vi "Register to IncomingMessages.vi"(8 "error in":errorcluster, 11 "Actor Class":T1) -> (0 "error out":errorcluster, 3 "Incoming Messages":refnum<event-registration>)   [LabVIEW 2013]
uses:
  Actor Private Data.ctl
  <vilib>/LabVIEW Open Source Project/MQTT Client/Client class/Client.lvclass
  Actor Private Events -- cluster.ctl
  Payload -- cluster.ctl
  <vilib>/LabVIEW Open Source Project/MQTT Client/Client class/Public Events -- cluster.ctl
  <vilib>/LabVIEW Open Source Project/MQTT Control Packets/Control Packets/CONNACK/Connect Return Code -- enum.ctl
  <vilib>/LabVIEW Open Source Project/MQTT Control Packets/Control Packets/PUBLISH/PUBLISH.lvclass
  <vilib>/LabVIEW Open Source Project/MQTT Client/Client class/Client.lvclass/Client.ctl
  <vilib>/LabVIEW Open Source Project/MQTT Control Packets/Control Packets/CONNACK/CONNACK.lvclass
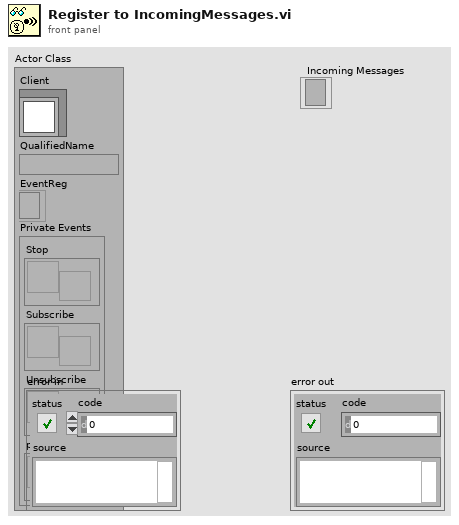
[diagram p1: front panel]
types:
  T1 = typedef "Actor Private Data.ctl" = cluster{"Client":refnum<class "Client.lvclass">, "QualifiedName":string, "EventReg":refnum<event-registration>, "Private Events":T2}
  T2 = typedef "Actor Private Events -- cluster.ctl" = cluster{"Stop":refnum<user-event>, "Subscribe":refnum<user-event>, "Unsubscribe":refnum<user-event>, "publish":refnum<user-event>}
  T3 = typedef "MQTT Client.lvlib/Client.lvclass/Public Events -- cluster.ctl" = cluster{"Connection Status":refnum<user-event>, "Connected":refnum<user-event>, "Application Message":refnum<user-event>}
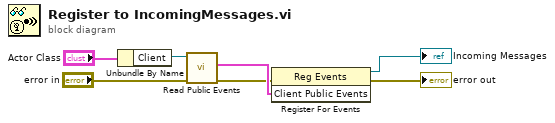
[diagram p0: block diagram]
diagram:
  n1 = Unbundle By Name("Actor Class") -> ("Client"=w6:refnum<class "Client.lvclass">)
  n2 = call <vilib>:"Read Public Events.vi"("error in (no error)"="error in", "Client in"=w6) -> ("error out"=w3:errorcluster, "Client Public Events"=w5:T3)  [unwired: 7 in, 1 out]
  n3 = register-events(error in=w3, w5) -> (reference out=→"Incoming Messages":refnum<event-registration>, error out=→"error out":errorcluster)  [unwired: 1 in]
